vi "setWFMQueue.vi"(4 "REF_Y":waveform(dbl)[](array[waveform]), 6 "REF_X":waveform(dbl)[](array[waveform]), 8 "error in (no error)":errorcluster, 10 "AO":waveform(dbl)[](array[waveform]), 11 "DAQmx in":refnum<class "DAQmx.lvclass">) -> (0 "error out":errorcluster, 3 "DAQmx out":refnum<class "DAQmx.lvclass">)   [LabVIEW 2019, in "DAQmx.lvclass"]
uses:
  DAQmx.lvclass
  DAQmx.lvclass/DAQmx.ctl
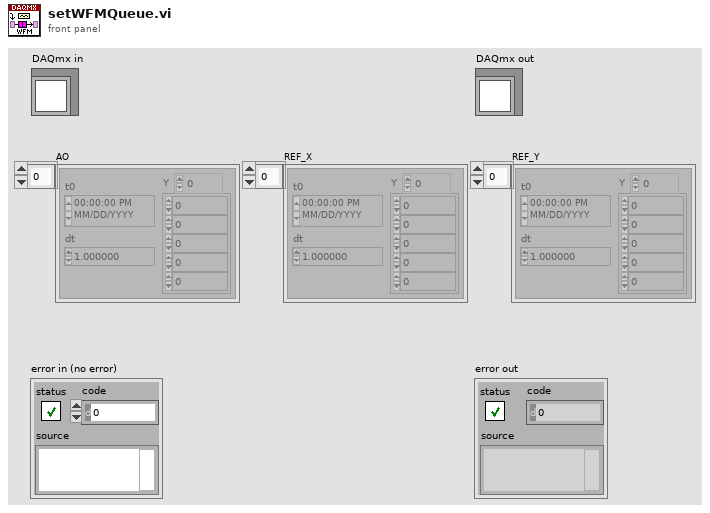
[diagram p1: front panel]
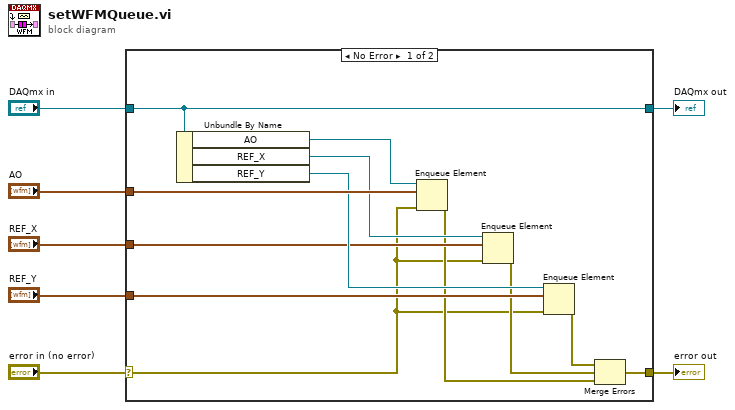
[diagram p0: block diagram]
diagram:
  n1 = case shown="No Error" "error in (no error)" {
    selector: "error in (no error)" -> [w9 w21]
    tunnel: [w10 w21] -> w6
    tunnel: [w19 w20] -> w4
    tunnel: "DAQmx in" -> [w19 w20]
    tunnel: "AO" -> [w18 _]
    tunnel: "REF_X" -> [w15 _]
    tunnel: "REF_Y" -> [w14 _]
    frame No Error {
      n2 = Unbundle By Name(w19) -> ("AO"=w8:refnum<queue>, "REF_X"=w17:refnum<queue>, "REF_Y"=w16:refnum<queue>)
      n3 = Enqueue Element(queue=w8, element=w18, error in (no error)=w9) -> (error out=w11:errorcluster)  [unwired: 1 in, 2 out]
      n4 = Enqueue Element(queue=w17, element=w15, error in (no error)=w9) -> (error out=w13:errorcluster)  [unwired: 1 in, 2 out]
      n5 = Enqueue Element(queue=w16, element=w14, error in (no error)=w9) -> (error out=w12:errorcluster)  [unwired: 1 in, 2 out]
      n6 = Merge Errors(w12, w13, w11) -> (w10:errorcluster)
    }
    frame Error {
    }
  }
  "error out" <- w6
  "DAQmx out" <- w4
